vi "CSM - State Table - DebugTool.vi"() -> ()   [LabVIEW 2014]
uses:
  _Support/Typedef/_CSM_GlobalLog_MSG.ctl
  _Support/Typedef/_CSM_GlobalLog_MSG_TYPE.ctl
  _Polymophic/Add State(s) to Queue By BOOL(Element).vi
  _Support/GlobalEvent/FGV-GlobalEventRef.vi
  <resource>/dialog/lvconfig.llb/LV Config Write Numeric (I32).vi
  <resource>/dialog/lvconfig.llb/LV Config Read Numeric (I32).vi
  _Support/csm-tool-support.lvlib
  Communicable State Machine.lvlib
panel:
  in  "Clear JKISM":bool
  out "Dashboard":T1(array[cluster])
  out "Table Control":string[][](table)
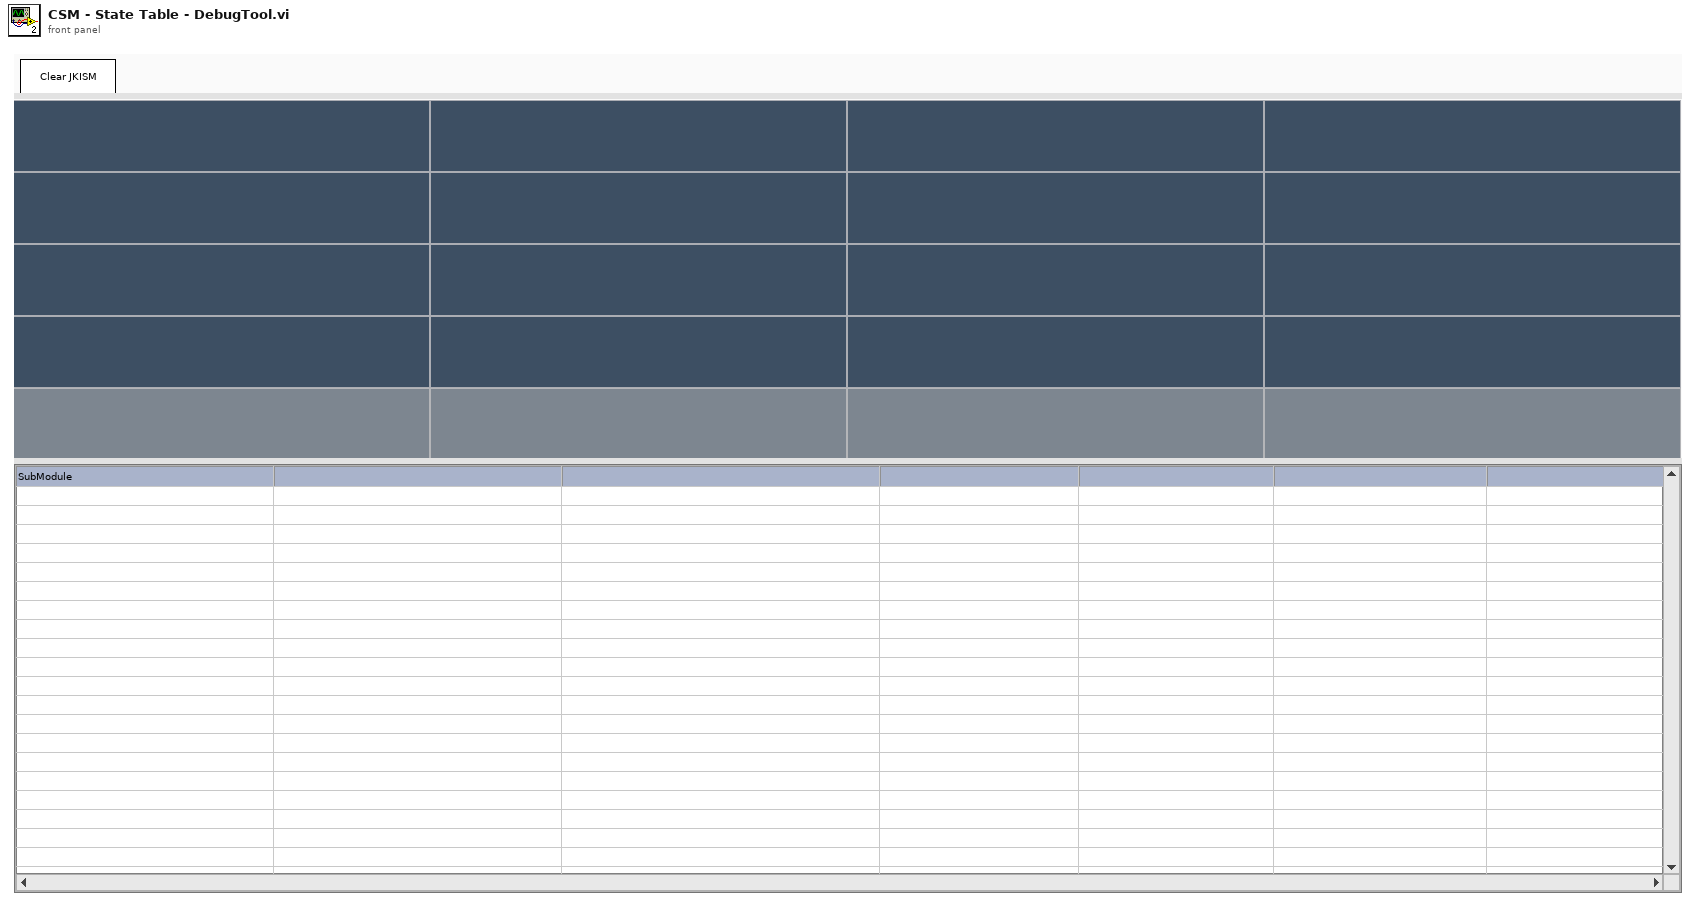
[diagram p1: front panel]
types:
  T1 = cluster{"Label":string, "Value":string, "String":string}[][]
  T2 = enum32{"Invalid", "Standard", "Closed", "Hidden", "Minimized", "Maximized"}
  T3 = enum32{"invalid app kind", "Development System", "Run Time System", "Student Edition", "Embedded LabVIEW", "Evaluation", "Custom"}
  T4 = typedef "Communicable State Machine.lvlib/_CSM_GlobalLog_MSG.ctl" = cluster{"Name(\"\" to use uuid)":string, "Current State":string, "Arguments":string, "Argument - State":string, "From Who":string, "Complete(T)/Start(F)":bool, "Type":T5}
  T5 = typedef "Communicable State Machine.lvlib/_CSM_GlobalLog_MSG_TYPE.ctl" = enum16{"User Log", "State Change", "Status", "Interrupt", "Register", "Unregister"}
  T6 = cluster{"Label":string, "Value":string, "String":string}
  T7 = cluster{"Core":cluster{"Current VI Reference":refnum<vi>, "Close Panel on Exit?":bool}, "Global-DataTable":string[][], "NumCols":i16, "NumRows":i16, "CSM Global Log Event":refnum<user-event>, "Log":T4, "JKISM Names":string[]}
  T8 = cluster{"Current VI Reference":refnum<vi>, "Close Panel on Exit?":bool}
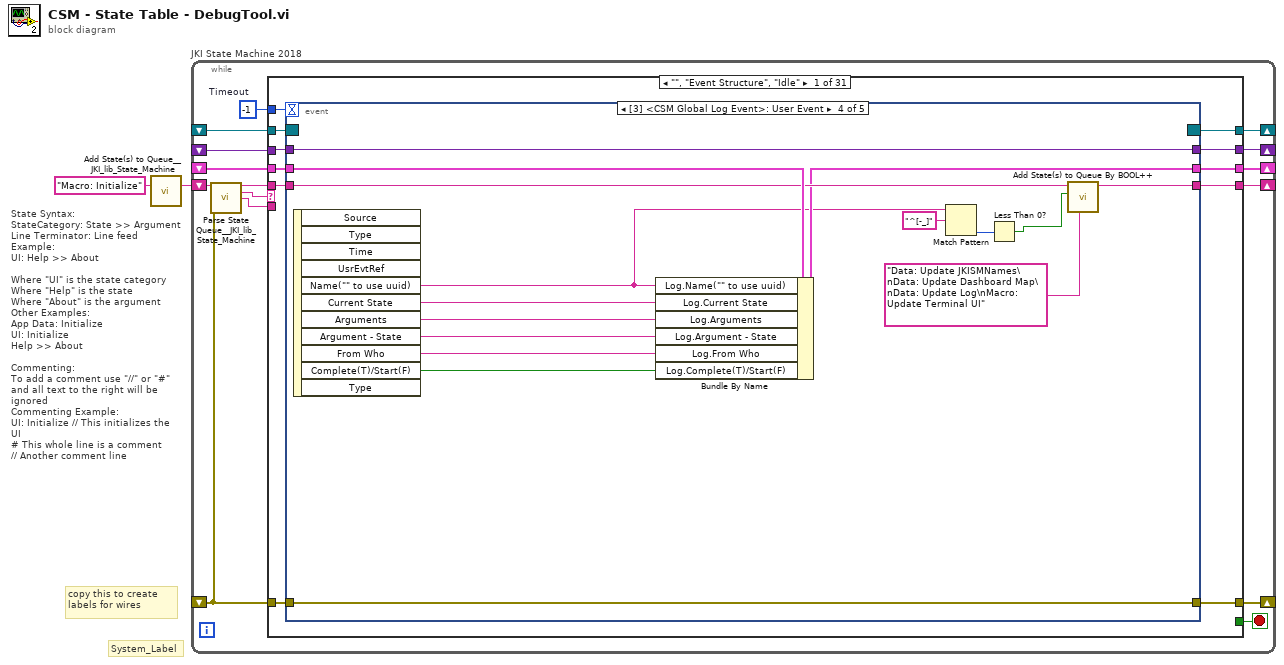
[diagram p0: block diagram]
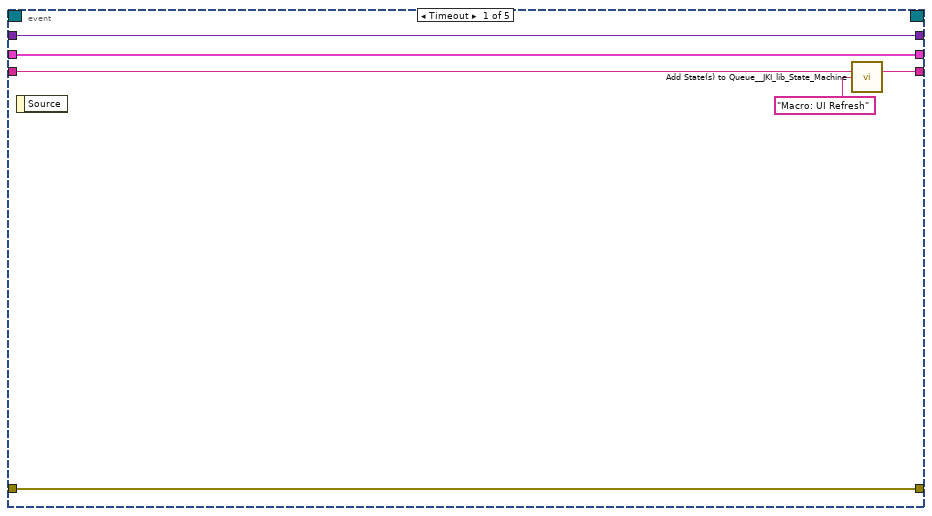
[diagram p2: hidden frame]
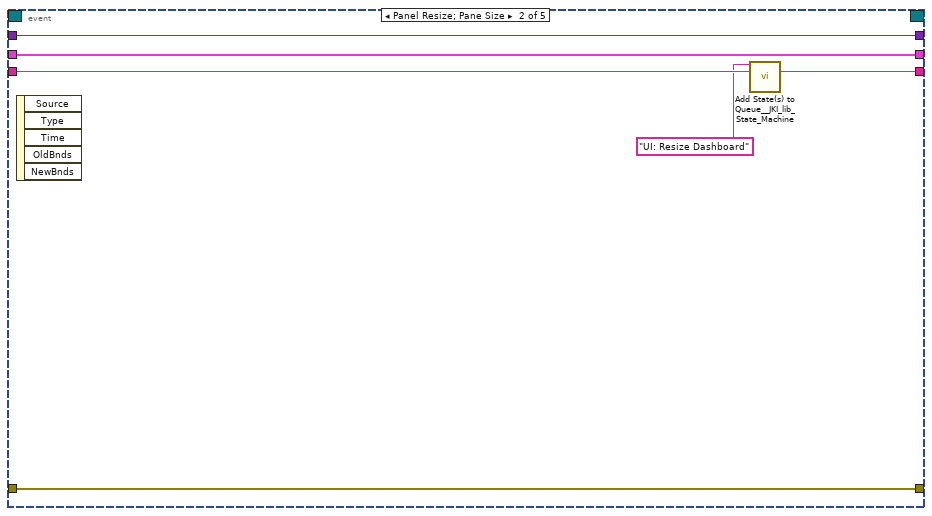
[diagram p3: hidden frame]
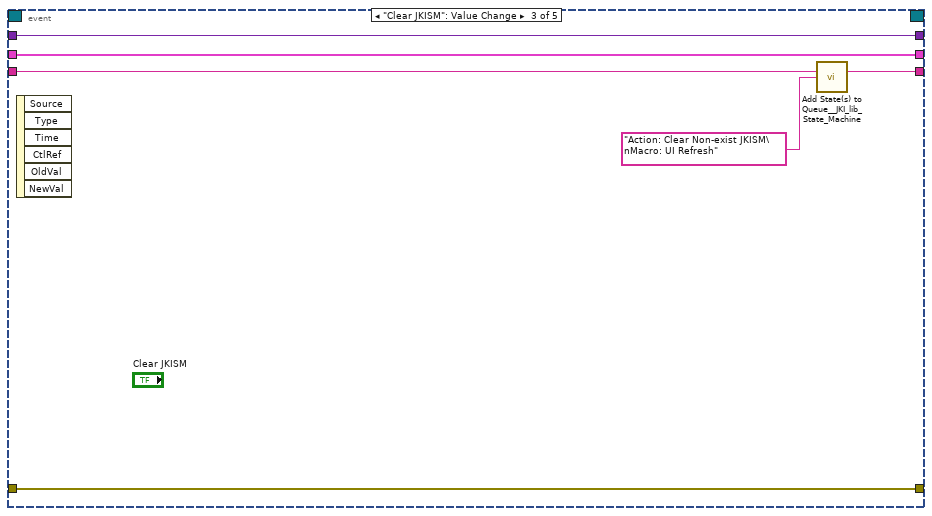
[diagram p4: hidden frame]
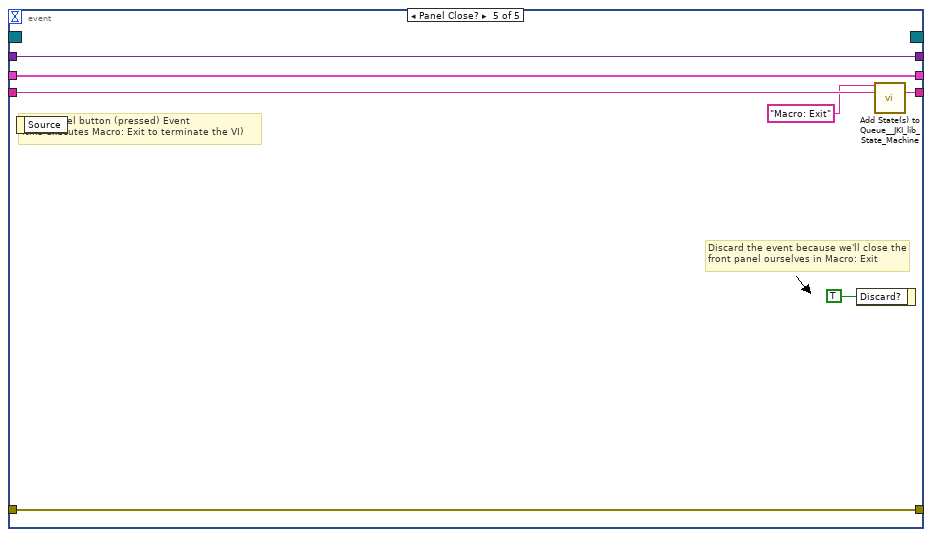
[diagram p5: hidden frame]
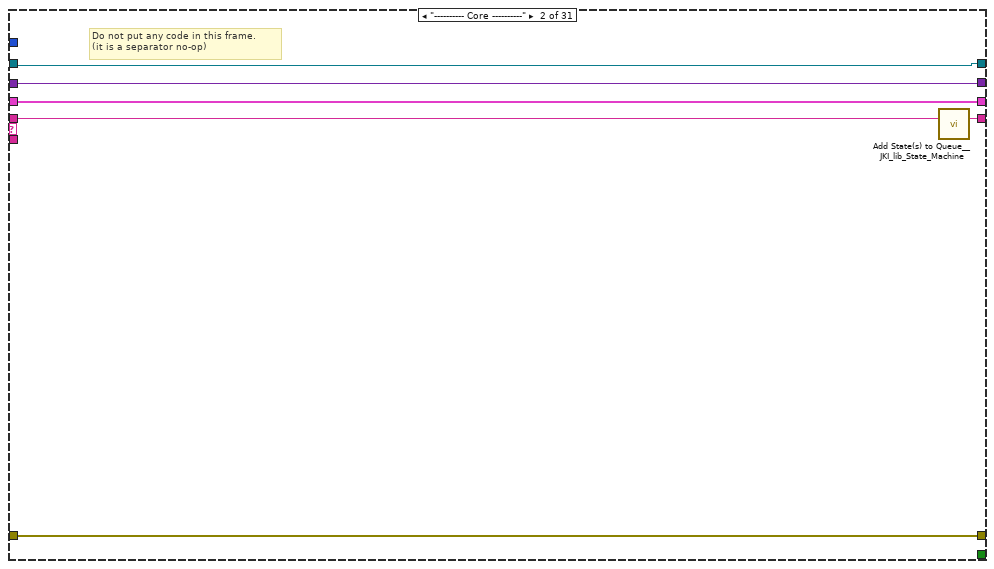
[diagram p6: hidden frame]
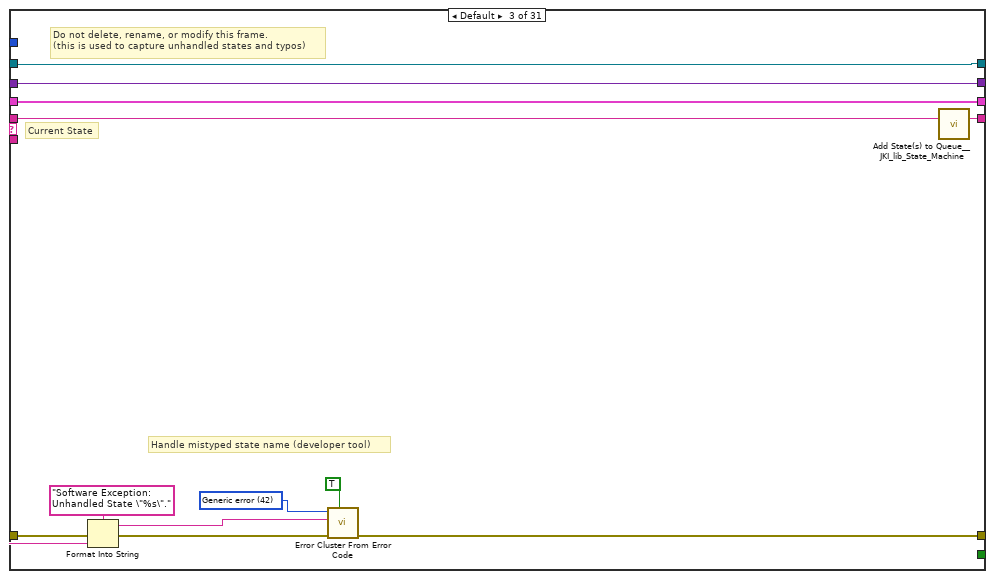
[diagram p7: hidden frame]
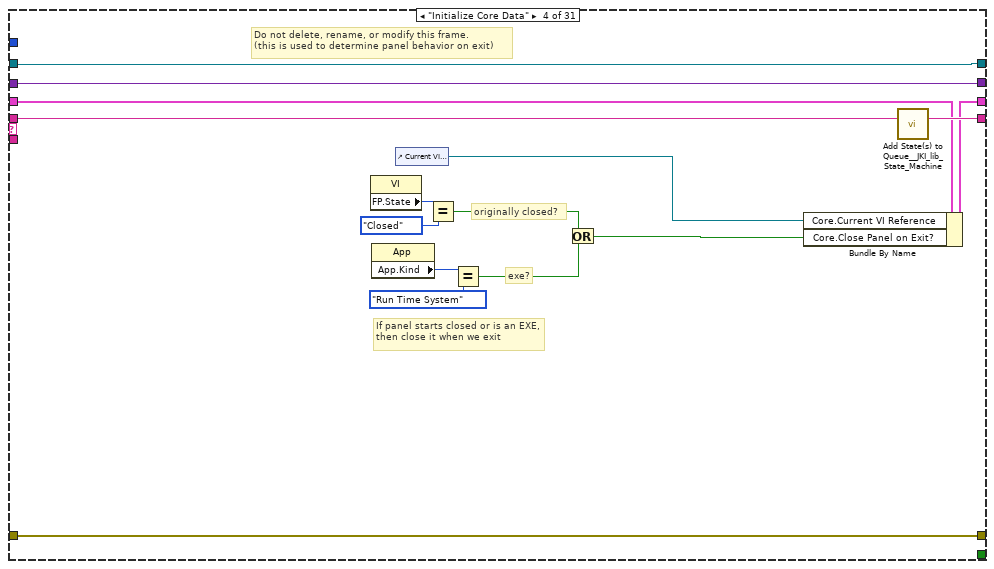
[diagram p8: hidden frame]
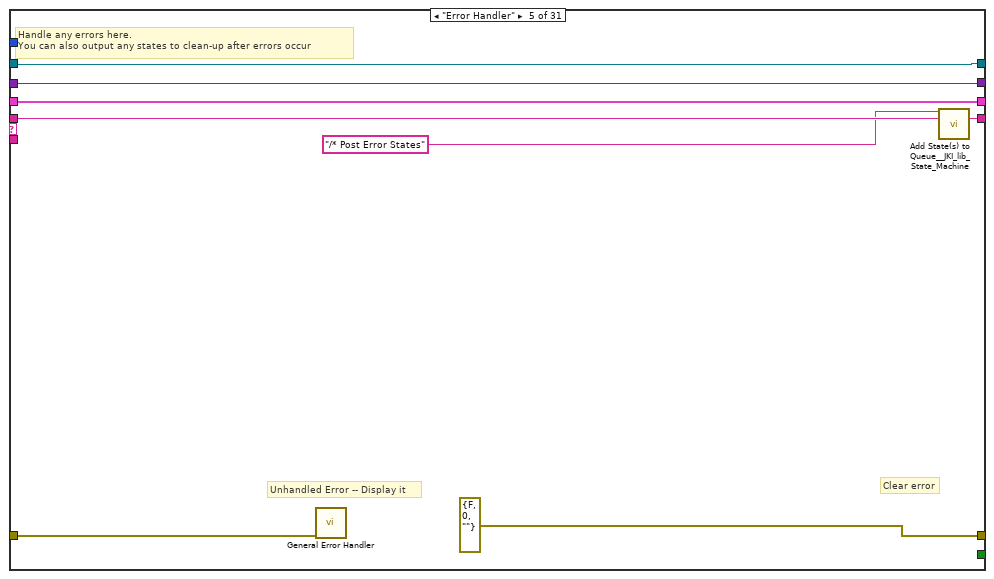
[diagram p9: hidden frame]
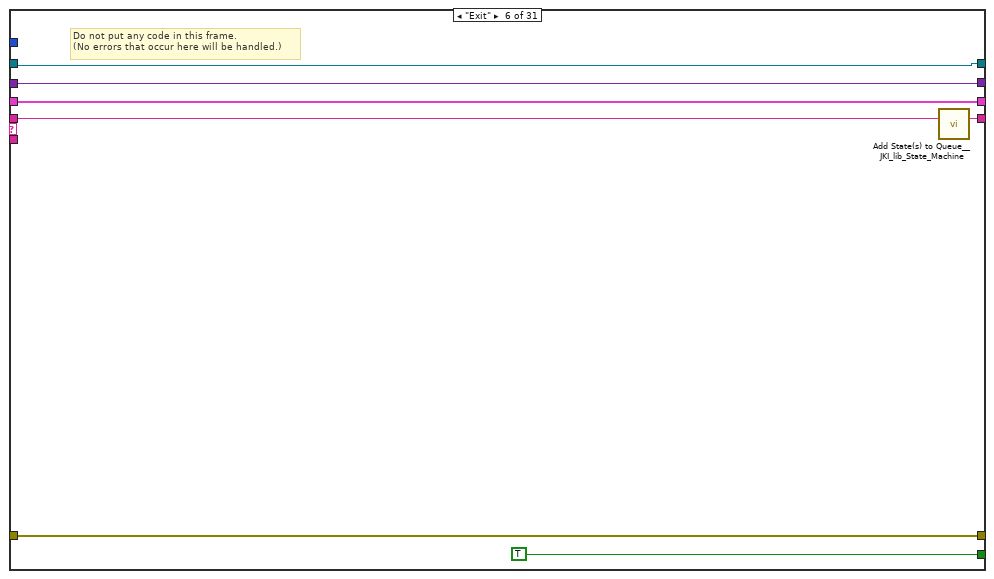
[diagram p10: hidden frame]
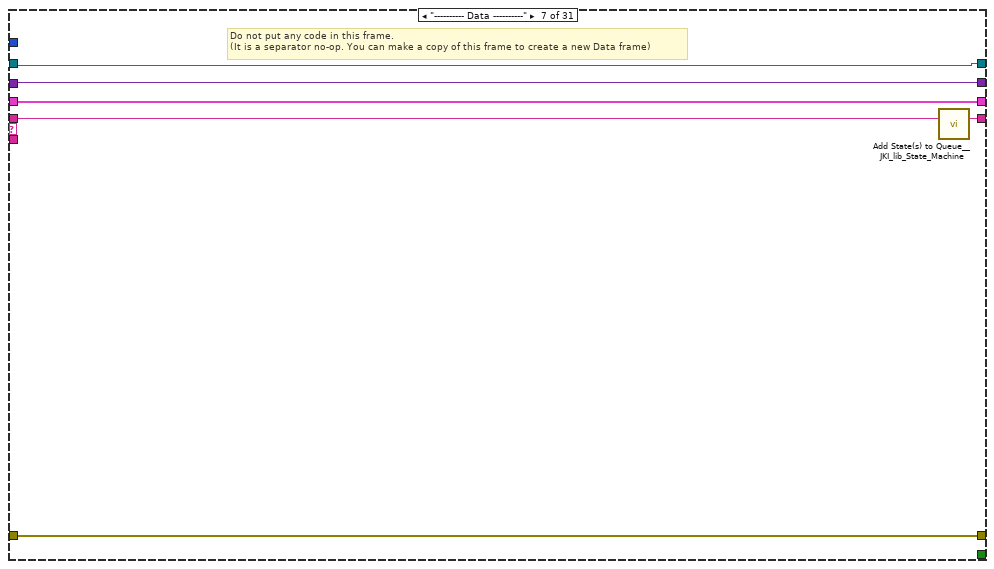
[diagram p11: hidden frame]
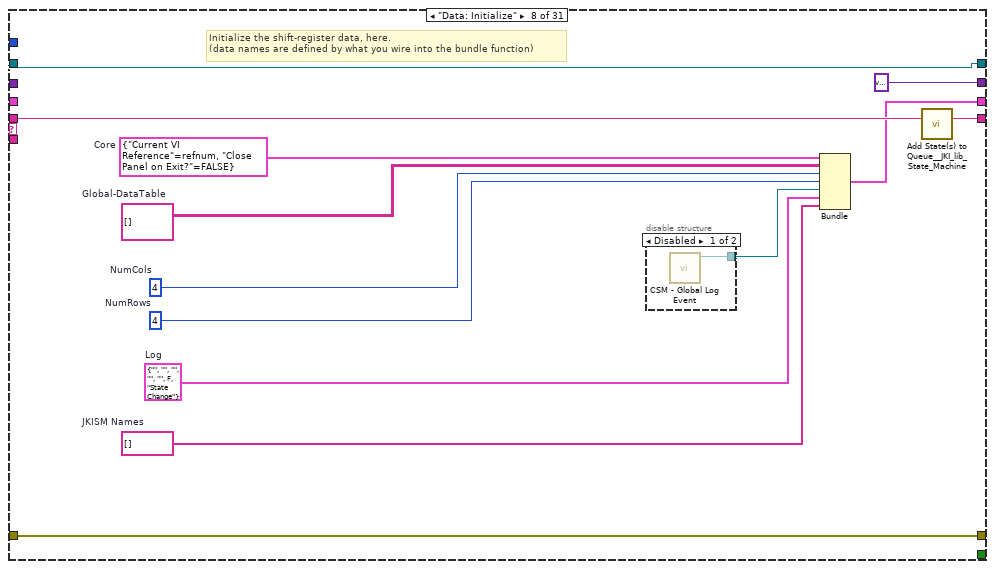
[diagram p12: hidden frame]
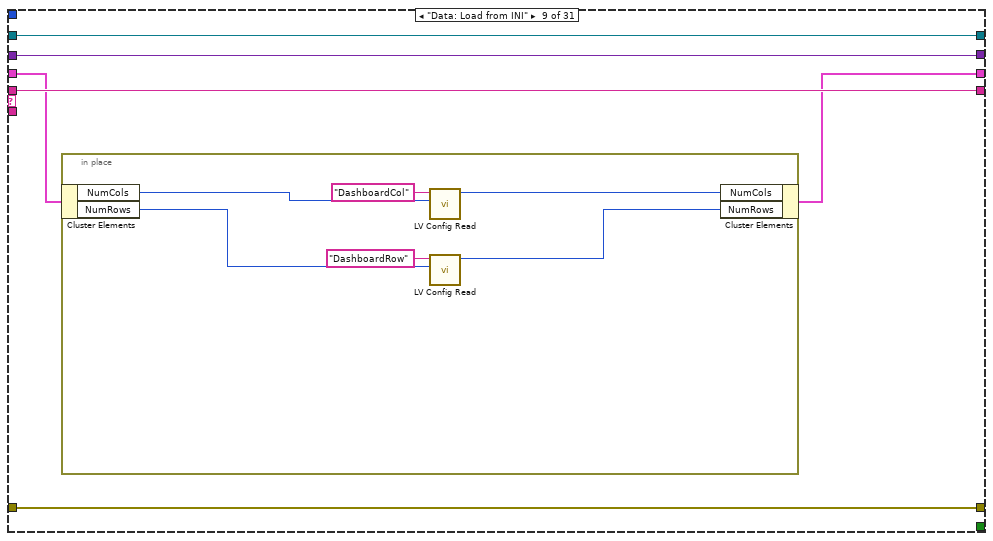
[diagram p14: hidden frame]
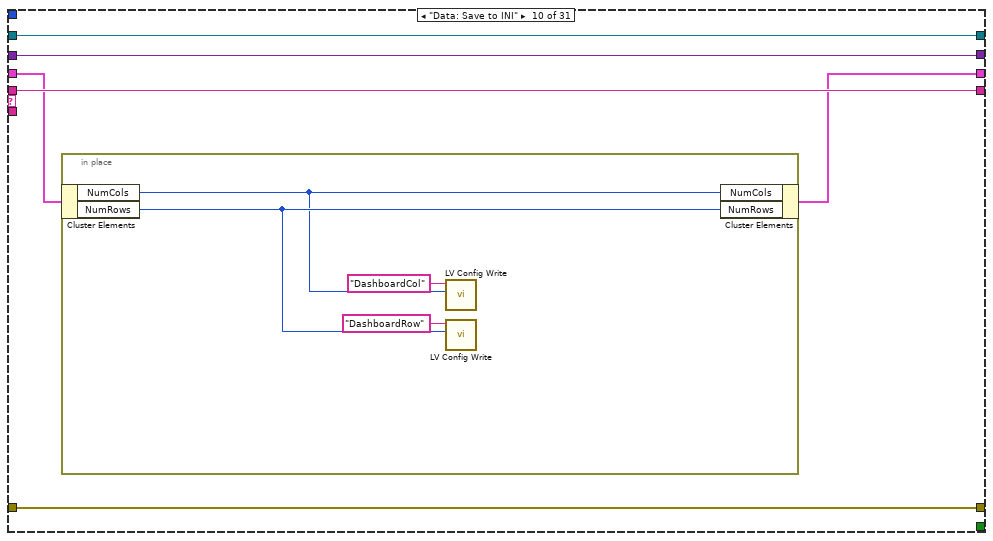
[diagram p15: hidden frame]
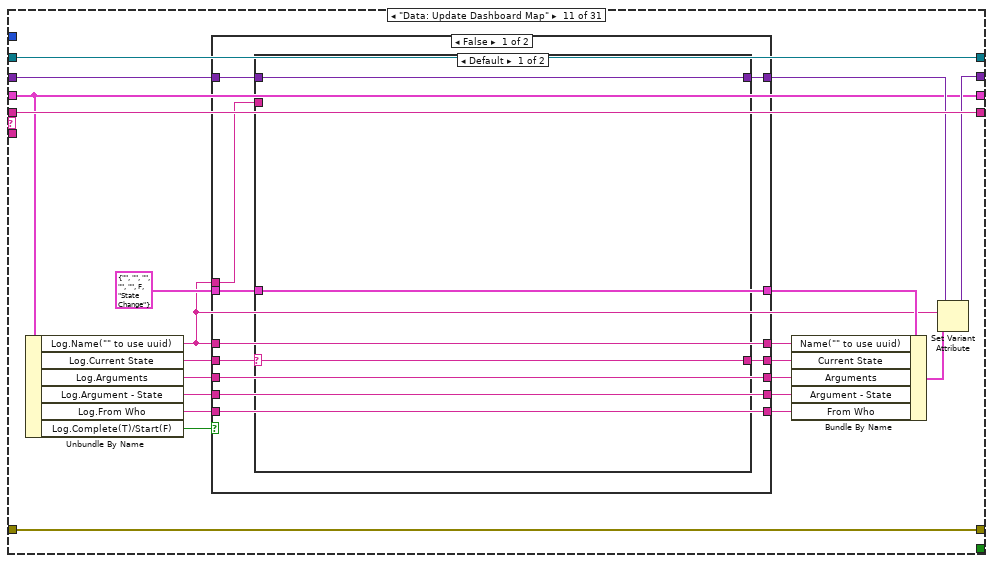
[diagram p16: hidden frame]
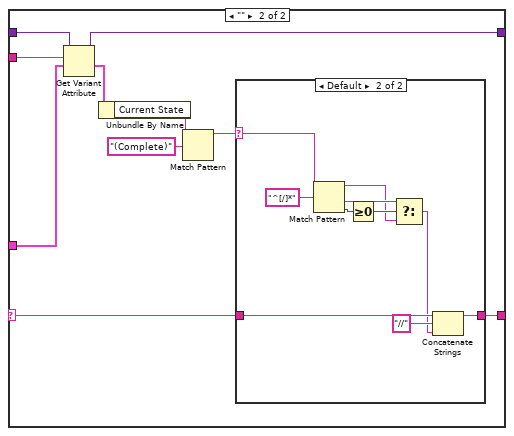
[diagram p17: hidden frame]
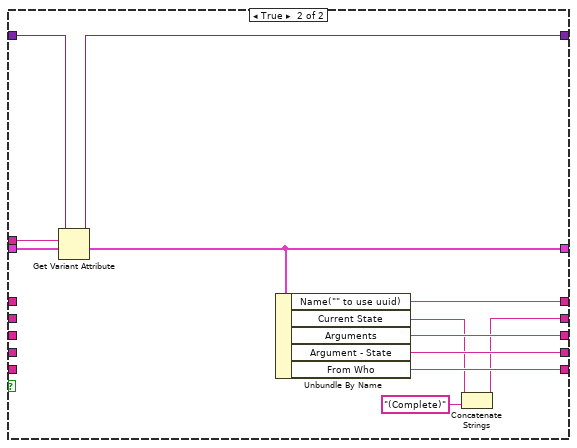
[diagram p19: hidden frame]
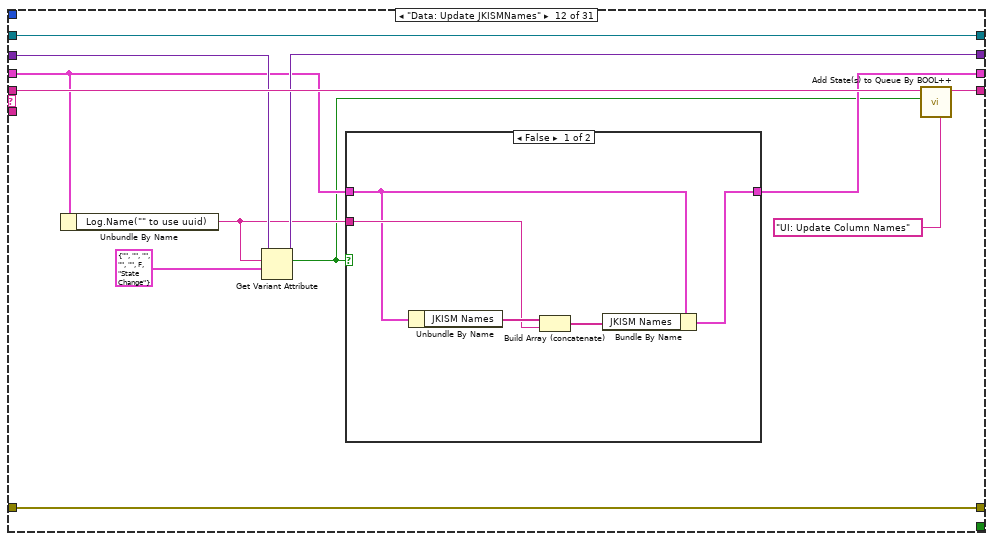
[diagram p20: hidden frame]
diagram:
  # "State Syntax:\nStateCategory: State >> Argument\nLine Terminator: Line feed\nExample:\nUI: Help >> About\n\nWhere \"UI\" is the state category\nWhere \"Help\" is the state\nWhere \"About\" is the argument\nOther Examples:\nApp Data: Initialize\nUI: Initialize\nHelp >> About\n\nCommenting:\nTo add a comment use \"//\" or \"#\" and all text to the right will be ignored\nCommenting Example:\nUI: Initialize // This initializes the UI\n# This whole line is a comment\n// Another comment line"
  # "copy this to create labels for wires"
  # "System_Label"
  n1 = call <vilib>:"Add State(s) to Queue__JKI_lib_State_Machine.vi"("State(s) in (\"\")"="Macro: Initialize") -> ("States Out"=w1:string)  [unwired: 14 in]
  n2 = while "JKI State Machine 2018" {
    shift-right: [w10] -> _
    shift-left: _ -> [w9]
    shift-right: [w13] -> _
    shift-left: _ -> [w7]
    shift-right: [w12] -> _
    shift-left: w1 -> [w14]
    shift-right: [w6] -> _
    shift-left: _ -> [w5]
    shift-right: [w4] -> _
    shift-left: _ -> [w3]
    stop <- w11 stop-if-true
    w8 = -1  # Timeout
    n3 = call <vilib>:"Parse State Queue__JKI_lib_State_Machine.vi"("State Queue"=w14, "Error In (no error)"=w7) -> ("Remaining States"=w16:string, "Current State"=w17:string, "Arguments"=w15:string)  [unwired: 11 in]
    n4 = case shown="\"\", \"Event Structure\", \"Idle\"" w17 {
      selector: w17 -> [_ _ w78 _ _ _ _ _ _ _ _ _ _ _ _ _ _ _ _ _ _ _ _ _ _ _ _ _ _ _ _]
      tunnel: w16 -> [w28 w75 w82 w103 w111 w118 w124 w137 w143 w155 w180 w237 w260 w283 w289 w298 w310 w323 w400 w415 w426 w431 w439 w447 w454 w461 w469 w476 w489 w493 w504]
      tunnel: w15 -> [_ _ _ _ _ _ _ _ _ _ _ _ _ _ _ _ w305 w317 _ _ _ _ _ _ _ _ _ _ _ _ _]
      tunnel: w9 -> [w26 w72 w80 w96 w108 w116 w121 _ w142 w154 w167 w231 w256 w278 w286 w294 w308 w319 w396 w412 w423 w430 w438 w443 w451 w458 w464 w473 w486 w492 w503]
      tunnel: [w25 w73 w84 w100 errorcluster {"status"=FALSE, "code"=0, "source"=""} ("error out") w115 w122 w133 w144 w156 w181 w238 w261 w277 w287 w296 w306 w320 w397 w413 w427 w432 w440 w448 w452 w459 w467 w474 w487 w494 w505] -> w13
      tunnel: w7 -> [w24 w73 w83 w100 w107 w115 w122 w133 w144 w156 w181 w238 w261 w280 w287 w296 w307 w321 _ w413 w427 w432 w440 w448 w452 w459 w467 w474 w487 w494 w505]
      tunnel: [w27 w74 w81 w102 w110 w117 w123 w136 w143 w155 w180 w229 w260 w282 w288 w297 w309 w322 w399 w414 w426 w431 w439 w447 w453 w460 w468 w475 w488 w493 w504] -> w12
      tunnel: [_ _ _ _ _ TRUE _ _ _ _ _ _ _ _ _ _ _ _ _ _ _ _ _ _ _ _ _ _ _ _ _] -> w11
      tunnel: [w23 w72 w80 w101 w108 w116 w121 w135 w141 w153 w167 w230 w256 w278 w286 w294 w308 w319 w396 w412 w423 w430 w434 w443 w451 w458 w464 w473 w486 w492 w503] -> w10
      tunnel: w8 -> [w22 _ _ _ _ _ _ _ _ _ _ _ _ _ _ _ _ _ _ _ _ _ _ _ _ _ _ _ _ _ _]
      tunnel: [w20 w71 w77 w90 w105 w113 w120 variant w140 w152 w168 w235 w257 w276 w285 w291 w304 w316 w393 w407 w425 w429 w437 w446 w450 w456 w463 w471 w479 w491 w499] -> w6
      tunnel: w5 -> [w21 w71 w77 w90 w105 w113 w120 _ w140 w152 w169 w233 w258 w276 w285 w291 w304 w316 w393 w406 w425 w429 w437 w446 w450 w456 w463 w471 w479 w491 w501]
      tunnel: [w18 w70 w76 w89 w104 w112 w119 w128 w139 w151 w179 w236 w259 w275 w284 w290 w303 w315 w392 w403 w424 w428 w435 w445 w449 w455 w462 w470 w478 w490 w502] -> w4
      tunnel: w3 -> [w19 w70 w76 w89 w104 w112 w119 w128 w139 w151 w179 w236 w259 w275 w284 w290 w303 w315 w392 w403 w424 w428 _ w445 w449 w455 w462 w470 w478 w490 w502]
      frame "", "Event Structure", "Idle" {
        n5 = event shown="[3] <CSM Global Log Event>: User Event" {
          selector: w19 -> [_ _ _ _ _]
          dyn-events: [_ _ _ _ _] -> w18
          timeout: w22 -> [_ _ _ _ _]
          tunnel: w28 -> [w34 w37 w43 w57 w69]
          tunnel: [w33 w38 w42 w61 w68] -> w27
          tunnel: w26 -> [w31 w39 w45 w58 w67]
          tunnel: [w32 w40 w46 w62 w64] -> w25
          tunnel: w24 -> [w32 w40 w46 w62 w64]
          tunnel: [w31 w39 w45 w56 w67] -> w23
          tunnel: w21 -> [w29 w35 w44 w59 w63]
          tunnel: [w29 w35 w44 w59 w63] -> w20
          event Timeout {
            n6 = event-data() -> ()  [unwired: 1 in, 1 out]
            n7 = call <vilib>:"Add State(s) to Queue__JKI_lib_State_Machine.vi"("State(s) in (\"\")"=w34, "State(s) at Back (\"\")"="Macro: UI Refresh" ("State(s) in Front (\"\")")) -> ("States Out"=w33:string)  [unwired: 13 in]
          }
          event Panel Resize; Pane Size {
            n8 = event-data() -> ()  [unwired: 1 in, 5 out]
            n9 = call <vilib>:"Add State(s) to Queue__JKI_lib_State_Machine.vi"("State(s) in Front (\"\")"="UI: Resize Dashboard" ("State(s) in Front (\"\")"), "State(s) in (\"\")"=w37) -> ("States Out"=w38:string)  [unwired: 13 in]
          }
          event "Clear JKISM": Value Change {
            n10 = event-data() -> ()  [unwired: 1 in, 6 out]
            n11 = call <vilib>:"Add State(s) to Queue__JKI_lib_State_Machine.vi"("State(s) in (\"\")"=w43, "State(s) at Back (\"\")"="Action: Clear Non-exist JKISM\nMacro: UI Refresh" ("State(s) at Back (\"\")")) -> ("States Out"=w42:string)  [unwired: 13 in]
          }
          event User Event {
            n12 = event-data() -> ("Name(\"\" to use uuid)"=w50:string, "Current State"=w51:string, "Arguments"=w52:string, "Argument - State"=w53:string, "From Who"=w54:string, "Complete(T)/Start(F)"=w55:bool)  [unwired: 1 in, 5 out]
            n13 = Bundle By Name(cluster=w58, "Log.Name(\"\" to use uuid)"=w50, "Log.Current State"=w51, "Log.Arguments"=w52, "Log.Argument - State"=w53, "Log.From Who"=w54, "Log.Complete(T)/Start(F)"=w55) -> (w56:T7)
            n14 = Match Pattern(string=w50, regular expression="^[-_]") -> (offset past match=w48:i32)  [unwired: 1 in, 3 out]
            n15 = Less Than 0?(x=w48) -> (x < 0?=w47:bool)
            n16 = call-poly "Add State(s) to Queue By BOOL++.vi"("TRUE(\"\")"="Data: Update JKISMNames\nData: Update Dashboard Map\nData: Update Log\nMacro: Update Terminal UI" ("State(s) at Back (\"\")"), "Bool"=w47, "State Queue(\"\")"=w57) -> ("State Queue Out"=w61:string)  [unwired: 8 in]
          }
          event Panel Close? {
            # "Discard the event because we'll close the front panel ourselves in Macro: Exit"
            # "Close Panel button (pressed) Event\n(this executes Macro: Exit to terminate the VI)"
            n17 = event-data() -> ()  [unwired: 1 in, 1 out]
            n18 = event-data("Discard?"=TRUE) -> ()  [unwired: 1 in, 1 out]
            n19 = call <vilib>:"Add State(s) to Queue__JKI_lib_State_Machine.vi"("State(s) in Front (\"\")"="Macro: Exit", "State(s) in (\"\")"=w69) -> ("States Out"=w68:string)  [unwired: 13 in]
          }
        }
      }
      frame "---------- Core ----------" {
        # "Do not put any code in this frame.\n(it is a separator no-op)"
        n20 = call <vilib>:"Add State(s) to Queue__JKI_lib_State_Machine.vi"("State(s) in (\"\")"=w75) -> ("States Out"=w74:string)  [unwired: 14 in]
      }
      frame Default {
        w87 = 42 items=["No error", "Argument error", "Memory is full", "Out of zone", "End of file", "File already open", "Generic file I/O error", "File not found", "File permission error", "Disk is full", "Duplicate path", "Too many files open", "System feature not enabled", "Resource file not found", "Cannot add resource", "Resource not found", "Image not found", "Image memory error", "Pen does not exist", "Config type invalid", "Config token not found", "Config parse error", "Config memory error", "Bad external code format", "Bad external code offset", "External code not present", "Null window", "Destroy window error", "Null menu", "Print aborted", "Bad print record", "Print driver error", "Windows error during printing", "Memory error during printing", "Print dialog error", "Generic print error", "Invalid device refnum", "Device not found", "Device parameter error", "Device unit error", "Cannot open device", "Device call aborted", "Generic error", "Cancelled by user", "Object ID too low", "Object ID too high", "Object not in heap", "Unknown heap", "Unknown object (invalid DefProc)", "Unknown object (DefProc not in table)", "Message out of range", "Invalid (null) method", "Unknown message", "Manager call not supported", "Bad address", "Network operation in progress", "Network operation timed out", "Connection is busy", "Network attribute not supported", "Network error", "Address in use", "System out of memory", "Connection aborted", "Connection refused", "Not connected", "Already connected", "Connection closed", "Initialization error (interapplication manager)", "Bad occurrence", "Wait on unbound occurrence handler", "Occurrence queue overflow", "Datalog type conflict", "Unused", "Unrecognized type (interapplication manager)", "Memory corrupt", "Failed to make temporary DLL", "Old CIN version", "Drag socket not found", "Failed to load drop-object", "Failed to register OLE object", "Failed to release OLE object", "Format specifier type mismatch", "Unknown format specifier", "Too few format specifiers", "Too many format specifiers", "Scan failed", "Newer CIN version", "Error converting to variant", "Runtime menu error", "Password tampered", "Variant attribute not found", "Incompatible variant data type", "Event data is not available", "Event Store is not present", "Occurrence is not found", "Event Queue is not created", "Event info is not available", "Refnum passed is NULL", "Error retrieving Class GUID", "Error retrieving CoClass GUID", "Error retrieving TypeLib GUID.", "Bad built application magic bytes.", "Specific driver is different from the specific driver associated with the Logical Name.", "There is no session opened to the class driver.", "Max Error", "MAX - Error with config objects", "MAX - Error loading configuration", "MAX - Group not supported"]
        # "Current State"
        # "Do not delete, rename, or modify this frame.\n(this is used to capture unhandled states and typos)"
        # "Handle mistyped state name (developer tool)"
        n21 = Format Into String(format string="Software Exception: Unhandled State \"%s\"." ("message"), error in=w83, w78) -> (resulting string=w86:string, error out=w85:errorcluster)  [unwired: 1 in]
        n22 = call <vilib>:"Error Cluster From Error Code.vi"("show call chain? (False)"=TRUE, "error in (no error)"=w85, "error message (\"\")"=w86, "error code (0)"=w87) -> ("error out"=w84:errorcluster)  [unwired: 5 in]
        n23 = call <vilib>:"Add State(s) to Queue__JKI_lib_State_Machine.vi"("State(s) in (\"\")"=w82) -> ("States Out"=w81:string)  [unwired: 14 in]
      }
      frame "Initialize Core Data" {
        # "Do not delete, rename, or modify this frame.\n(this is used to determine panel behavior on exit)"
        # "originally closed?"
        # "exe?"
        # "If panel starts closed or is an EXE, then close it when we exit"
        n24 = property class="VI"() -> ("FP.State"=w93:T2)  [unwired: 2 in, 2 out]
        n25 = property class="App"() -> ("App.Kind"=w99:T3)  [unwired: 2 in, 2 out]
        n26 = control-ref of="Current VI Reference"() -> (w94:refnum<vi>)
        n27 = Equal?(x=w93, y=T2."Closed" ("Front Panel Window:State")) -> (x = y?=w91:bool)
        n28 = Equal?(x=w99, y=T3."Run Time System" ("Application:Kind")) -> (x = y?=w97:bool)
        n29 = Or(x=w91, y=w97) -> (x .or. y?=w95:bool)
        n30 = Bundle By Name(cluster=w96, "Core.Current VI Reference"=w94, "Core.Close Panel on Exit?"=w95) -> (w101:T7)
        n31 = call <vilib>:"Add State(s) to Queue__JKI_lib_State_Machine.vi"("State(s) in (\"\")"=w103) -> ("States Out"=w102:string)  [unwired: 14 in]
      }
      frame "Error Handler" {
        # "Unhandled Error -- Display it"
        # "Handle any errors here.\nYou can also output any states to clean-up after errors occur"
        # "Clear error"
        n32 = call <vilib>:"General Error Handler.vi"("error in (no error)"=w107) -> ()  [unwired: 10 in, 5 out]
        n33 = call <vilib>:"Add State(s) to Queue__JKI_lib_State_Machine.vi"("State(s) in Front (\"\")"="/* Post Error States", "State(s) in (\"\")"=w111) -> ("States Out"=w110:string)  [unwired: 13 in]
      }
      frame "Exit" {
        # "Do not put any code in this frame.\n(No errors that occur here will be handled.)"
        n34 = call <vilib>:"Add State(s) to Queue__JKI_lib_State_Machine.vi"("State(s) in (\"\")"=w118) -> ("States Out"=w117:string)  [unwired: 14 in]
      }
      frame "---------- Data ----------" {
        # "Do not put any code in this frame.\n(It is a separator no-op. You can make a copy of this frame to create a new Data frame)"
        n35 = call <vilib>:"Add State(s) to Queue__JKI_lib_State_Machine.vi"("State(s) in (\"\")"=w124) -> ("States Out"=w123:string)  [unwired: 14 in]
      }
      frame "Data: Initialize" {
        w125 = string[] []  # JKISM Names
        w126 = T4 {"Name(\"\" to use uuid)"="", "Current State"="", "Arguments"="", "Argument - State"="", "From Who"="", "Complete(T)/Start(F)"=FALSE, "Type"=enum."State Change"}  # Log
        w131 = i16 4  # NumCols
        w130 = i16 4  # NumRows
        w132 = string[][] []  # Global-DataTable
        w134 = T8 {"Current VI Reference"=refnum, "Close Panel on Exit?"=FALSE}  # Core
        # "Initialize the shift-register data, here.\n(data names are defined by what you wire into the bundle function)"
        n36 = disable-structure shown="Disabled" {
          disable-tunnel: [w138 _] -> w127
          frame Disabled {
            n37 = call "CSM - Global Log Event.vi"() -> ("CSM Global Log Event"=w138:refnum<user-event>)  [unwired: 10 in, 1 out]
          }
          frame Enabled {
          }
        }
        n38 = Bundle("Core"=w134, "Global-DataTable"=w132, "NumCols"=w131, "NumRows"=w130, "CSM Global Log Event"=w127, "Log"=w126, "JKISM Names"=w125) -> (w135:T7)  [unwired: 1 in]
        n39 = call <vilib>:"Add State(s) to Queue__JKI_lib_State_Machine.vi"("State(s) in (\"\")"=w137) -> ("States Out"=w136:string)  [unwired: 14 in]
      }
      frame "Data: Load from INI" {
        n40 = in-place {
          n41 = in-place-cluster #1(w142) -> ("NumCols"=w146:i16, "NumRows"=w149:i16)
          n42 = call-poly <resource>:"LV Config Read.vi"("default value"=w146, "key"="DashboardCol") -> ("value"=w145:i32)  [unwired: 3 in, 2 out]
          n43 = call-poly <resource>:"LV Config Read.vi"("default value"=w149, "key"="DashboardRow") -> ("value"=w148:i32)  [unwired: 3 in, 2 out]
          n44 = in-place-cluster #1("NumCols"=w145, "NumRows"=w148) -> (w141:T7)
        }
      }
      frame "Data: Save to INI" {
        n45 = in-place {
          n46 = in-place-cluster #2(w154) -> ("NumCols"=w157:i16, "NumRows"=w158:i16)
          n47 = call-poly <resource>:"LV Config Write.vi"("value"=w157, "key"="DashboardCol") -> ()  [unwired: 5 in, 1 out]
          n48 = call-poly <resource>:"LV Config Write.vi"("value"=w158, "key"="DashboardRow") -> ()  [unwired: 5 in, 1 out]
          n49 = in-place-cluster #2("NumCols"=w157, "NumRows"=w158) -> (w153:T7)
        }
      }
      frame "Data: Update Dashboard Map" {
        n50 = Unbundle By Name(w167) -> ("Log.Name(\"\" to use uuid)"=w161:string, "Log.Current State"=w166:string, "Log.Arguments"=w165:string, "Log.Argument - State"=w164:string, "Log.From Who"=w163:string, "Log.Complete(T)/Start(F)"=w162:bool)
        n51 = case shown="False" w162 {
          tunnel: w169 -> [w187 w226]
          tunnel: [w186 w225] -> w177
          tunnel: T4 {"Name(\"\" to use uuid)"="", "Current State"="", "Arguments"="", "Argument - State"="", "From Who"="", "Complete(T)/Start(F)"=FALSE, "Type"=enum."State Change"} ("Cross JKI State Machine Data") -> [w184 w224]
          tunnel: w161 -> [w185 w223]
          tunnel: w163 -> [w191 _]
          tunnel: [w191 w222] -> w175
          tunnel: w164 -> [w190 _]
          tunnel: [w190 w221] -> w174
          tunnel: w165 -> [w189 _]
          tunnel: [w189 w220] -> w173
          tunnel: w166 -> [w183 _]
          tunnel: [w182 w215] -> w172
          tunnel: w161 -> [w188 _]
          tunnel: [w188 w217] -> w171
          tunnel: [w184 w218] -> w170
          frame False {
            n52 = case shown="Default" w183 {
              selector: w183 -> [w192 w195]
              tunnel: w187 -> [w193 w203]
              tunnel: [w193 w202] -> w186
              tunnel: w185 -> [_ w201]
              tunnel: w184 -> [_ w199]
              tunnel: [w192 w194] -> w182
              frame Default {
              }
              frame "" {
                n53 = Get Variant Attribute(Variant=w203, name=w201, default value (empty Variant)=w199) -> (duplicate Variant=w202:variant, value=w200:T4)  [unwired: 1 in, 2 out]
                n54 = Unbundle By Name(w200) -> ("Current State"=w198:string)
                n55 = Match Pattern(string=w198, regular expression="(Complete)") -> (before substring=w196:string)  [unwired: 1 in, 3 out]
                n56 = case shown="Default" w196 {
                  selector: w196 -> [_ w210]
                  tunnel: w195 -> [w204 w214]
                  tunnel: [w204 w213] -> w194
                  frame "" {
                  }
                  frame Default {
                    n57 = Match Pattern(string=w210, regular expression="^[/]*") -> (before substring=w205:string, after substring=w207:string, offset past match=w209:i32)  [unwired: 1 in, 1 out]
                    n58 = Greater Or Equal To 0?(x=w209) -> (x >= 0?=w208:bool)
                    n59 = Select(t=w207, s=w208, f=w205) -> (s? t:f=w206:string)
                    n60 = Concatenate Strings(w214, "//" ("string"), w206) -> (w213:string)
                  }
                }
              }
            }
          }
          frame True {
            n61 = Get Variant Attribute(Variant=w226, name=w223, default value (empty Variant)=w224) -> (duplicate Variant=w225:variant, value=w218:T4)  [unwired: 1 in, 2 out]
            n62 = Unbundle By Name(w218) -> ("Name(\"\" to use uuid)"=w217:string, "Current State"=w216:string, "Arguments"=w220:string, "Argument - State"=w221:string, "From Who"=w222:string)
            n63 = Concatenate Strings(w216, "(Complete)" ("string")) -> (w215:string)
          }
        }
        n64 = Bundle By Name(cluster=w170, "Name(\"\" to use uuid)"=w171, "Current State"=w172, "Arguments"=w173, "Argument - State"=w174, "From Who"=w175) -> (w178:T4)
        n65 = Set Variant Attribute(Variant=w177, name=w161, value=w178) -> (Variant out=w168:variant)  [unwired: 1 in, 2 out]
      }
      frame "Data: Update JKISMNames" {
        n66 = Unbundle By Name(w231) -> ("Log.Name(\"\" to use uuid)"=w232:string)
        n67 = Get Variant Attribute(Variant=w233, name=w232, default value (empty Variant)=T4 {"Name(\"\" to use uuid)"="", "Current State"="", "Arguments"="", "Argument - State"="", "From Who"="", "Complete(T)/Start(F)"=FALSE, "Type"=enum."State Change"} ("Cross JKI State Machine Data")) -> (duplicate Variant=w235:variant, found=w228:bool)  [unwired: 1 in, 2 out]
        n68 = case shown="False" w228 {
          tunnel: w231 -> [w241 w244]
          tunnel: w232 -> [w242 _]
          tunnel: [w239 w244] -> w230
          frame False {
            n69 = Unbundle By Name(w241) -> ("JKISM Names"=w243:string[])
            n70 = Build Array (concatenate)(w243, w242) -> (w240:string[])
            n71 = Bundle By Name(cluster=w241, "JKISM Names"=w240) -> (w239:T7)
          }
          frame True {
          }
        }
        n72 = call-poly "Add State(s) to Queue By BOOL++.vi"("False(\"\")"="UI: Update Column Names" ("TRUE(\"\")"), "Bool"=w228, "State Queue(\"\")"=w237) -> ("State Queue Out"=w229:string)  [unwired: 8 in]
      }
      frame "Data: Update Log" {
        n73 = Unbundle By Name(w256) -> ("JKISM Names"=w255:string[])
        n74 = for {
          shift-right: [w272] -> w257
          shift-left: w258 -> [w273]
          tunnel: w255 -> [w271] mode=indexing
          tunnel: [w269] -> w251 mode=indexing
          n75 = Get Variant Attribute(Variant=w273, name=w271, default value (empty Variant)=T4 {"Name(\"\" to use uuid)"="", "Current State"="", "Arguments"="", "Argument - State"="", "From Who"="", "Complete(T)/Start(F)"=FALSE, "Type"=enum."State Change"} ("Cross JKI State Machine Data")) -> (duplicate Variant=w272:variant, value=w270:T4)  [unwired: 1 in, 2 out]
          n76 = Unbundle By Name(w270) -> ("Current State"=w269:string)
        }
        n77 = Array Size(array=w251) -> (size(s)=w250:i32)
        n78 = feedback #3(string[][] []) -> (w249:string[][])
        n79 = Array Size(array=w249) -> (size(s)=w252:i32[])
        n80 = Index Array(array=w252) -> (element #1=w248:i32, element #2=w247:i32)  [unwired: 2 in]
        n81 = Greater?(x=w250, y=w247) -> (0:w245:bool)
        n82 = case shown="True" w245 {
          tunnel: w249 -> [w262 w268]
          tunnel: w248 -> [_ w266]
          tunnel: w247 -> [_ w264]
          tunnel: [w262 w263] -> w246
          frame False {
          }
          frame True {
            n83 = Initialize Array("" ("Current State"), w266) -> (w265:string[])
            n84 = Insert Into Array(array=w268, index (col)=w264, new element=w265) -> (w263:string[][])  [unwired: 1 in]
          }
        }
        n85 = Build Array (concatenate)(w251, w246) -> (w254:string[][])
        "Table Control" <- w254
        n86 = feedback-in #3(w254) -> ()
      }
      frame "Data: Cleanup" {
        # "Cleanup any data and references, here.\n(this is called automatically, by the Macro: Exit)"
        n87 = Unbundle By Name(w278) -> ("Core.Current VI Reference"=w281:refnum<vi>)
        n88 = Close Reference(reference=w281, error in (no error)=w280) -> (error out=w279:errorcluster)
        n89 = Merge Errors(w279) -> (w277:errorcluster)
        n90 = call <vilib>:"Add State(s) to Queue__JKI_lib_State_Machine.vi"("State(s) in (\"\")"=w283) -> ("States Out"=w282:string)  [unwired: 14 in]
      }
      frame "---------- UI ----------" {
        # "Do not put any code in this frame.\n(It is a separator no-op. You can make a copy of this frame to create a new UI frame)"
        n91 = call <vilib>:"Add State(s) to Queue__JKI_lib_State_Machine.vi"("State(s) in (\"\")"=w289) -> ("States Out"=w288:string)  [unwired: 14 in]
      }
      frame "UI: Initialize" {
        # "Initialize the User Interface, here.\n(this is called automatically, by the Macro: Init)"
        n92 = invoke class="VI" method="Default Vals.Reinit All"() -> (error out=w295:errorcluster)  [unwired: 3 in, 2 out]
        n93 = Unbundle By Name(w294) -> ("NumRows"=w293:i16, "NumCols"=w292:i16)
        n94 = flat-sequence {
          tunnel: w295 -> [_]
          tunnel: w293 -> [w300]
          tunnel: w292 -> [w299]
          frame #0 {
            n95 = Initialize Array(T6 {"Label"="", "Value"="", "String"=""} ("Dashboard"), w300, w299) -> (w301:T1)
            n96 = local write "Dashboard"(w301) -> ()
          }
        }
        n97 = call <vilib>:"Add State(s) to Queue__JKI_lib_State_Machine.vi"("State(s) in (\"\")"=w298) -> ("States Out"=w297:string)  [unwired: 14 in]
      }
      frame "UI: Cursor Set" {
        # "Argument"
        # "Set and Unset Cursor Busy.\n(Usage: \"UI: Cursor Set >> Busy|Idle\")"
        n98 = case shown="\"Idle\", Default" w305 {
          tunnel: w307 -> [w312 w314]
          tunnel: [w311 w313] -> w306
          frame "Idle", Default {
            n99 = call <vilib>:"Unset Busy.vi"("error in (no error)"=w312) -> ("error out"=w311:errorcluster)  [unwired: 10 in]
          }
          frame "Busy" {
            n100 = call <vilib>:"Set Busy.vi"("error in (no error)"=w314) -> ("error out"=w313:errorcluster)  [unwired: 9 in, 1 out]
          }
        }
        n101 = call <vilib>:"Add State(s) to Queue__JKI_lib_State_Machine.vi"("State(s) in (\"\")"=w310) -> ("States Out"=w309:string)  [unwired: 14 in]
      }
      frame "UI: Front Panel State" {
        # "Argument"
        # "Set Front Panel Open or Closed\n(Usage: \"UI: Front Panel State >> Open|Close\")"
        n102 = Unbundle By Name(w319) -> ("Core.Current VI Reference"=w318:refnum<vi>)
        n103 = case shown="\"Minimize\", \"Minimized\"" w317 {
          tunnel: w321 -> [w329 w344 w355 w368 w381]
          tunnel: [w331 w345 w357 w370 w383] -> w320
          tunnel: w318 -> [w330 w342 w356 w369 w382]
          frame "Open", "Standard", Default {
            w324 = T2."Standard" ("State")
            n104 = property class="VI"(reference=w330, error in=w329) -> (reference out=w327:refnum<vi>, error out=w328:errorcluster, "FP.State"=w326:T2)
            n105 = Not Equal?(x=w326, y=w324) -> (x != y?=w325:bool)
            n106 = case shown="True" w325 {
              tunnel: [w335 w337] -> w331
              tunnel: w328 -> [w334 w337]
              tunnel: w327 -> [w333 _]
              tunnel: w324 -> [w332 _]
              frame True {
                n107 = invoke class="VI" method="FP.Open"(reference=w333, error in=w334, "Activate"=TRUE, "State"=w332) -> (error out=w335:errorcluster)  [unwired: 1 in, 4 out]
              }
              frame False {
              }
            }
          }
          frame "Close", "Closed" {
            n108 = property class="VI"(reference=w342, error in=w344) -> (reference out=w341:refnum<vi>, error out=w343:errorcluster, "FP.State"=w339:T2)
            n109 = Not Equal?(x=w339, y=T2."Closed" ("Front Panel Window:State")) -> (x != y?=w338:bool)
            n110 = case shown="True" w338 {
              tunnel: [w346 w349] -> w345
              tunnel: w343 -> [w346 w348]
              tunnel: w341 -> [_ w347]
              frame False {
              }
              frame True {
                n111 = invoke class="VI" method="FP.Close"(reference=w347, error in=w348) -> (error out=w349:errorcluster)  [unwired: 1 in, 2 out]
              }
            }
          }
          frame "Hidden", "Hide" {
            w350 = T2."Hidden" ("State")
            n112 = property class="VI"(reference=w356, error in=w355) -> (reference out=w353:refnum<vi>, error out=w354:errorcluster, "FP.State"=w352:T2)
            n113 = Not Equal?(x=w352, y=w350) -> (x != y?=w351:bool)
            n114 = case shown="True" w351 {
              tunnel: [w361 w362] -> w357
              tunnel: w354 -> [w360 w362]
              tunnel: w353 -> [w359 _]
              tunnel: w350 -> [w358 _]
              frame True {
                n115 = invoke class="VI" method="FP.Open"(reference=w359, error in=w360, "State"=w358) -> (error out=w361:errorcluster)  [unwired: 2 in, 4 out]
              }
              frame False {
              }
            }
          }
          frame "Minimize", "Minimized" {
            w363 = T2."Minimized" ("State")
            n116 = property class="VI"(reference=w369, error in=w368) -> (reference out=w366:refnum<vi>, error out=w367:errorcluster, "FP.State"=w365:T2)
            n117 = Not Equal?(x=w365, y=w363) -> (x != y?=w364:bool)
            n118 = case shown="True" w364 {
              tunnel: [w374 w375] -> w370
              tunnel: w367 -> [w373 w375]
              tunnel: w366 -> [w372 _]
              tunnel: w363 -> [w371 _]
              frame True {
                n119 = invoke class="VI" method="FP.Open"(reference=w372, error in=w373, "State"=w371) -> (error out=w374:errorcluster)  [unwired: 2 in, 4 out]
              }
              frame False {
              }
            }
          }
          frame "Maximize", "Maximized" {
            w376 = T2."Maximized" ("State")
            n120 = property class="VI"(reference=w382, error in=w381) -> (reference out=w379:refnum<vi>, error out=w380:errorcluster, "FP.State"=w378:T2)
            n121 = Not Equal?(x=w378, y=w376) -> (x != y?=w377:bool)
            n122 = case shown="True" w377 {
              tunnel: [w387 w388] -> w383
              tunnel: w380 -> [w386 w388]
              tunnel: w379 -> [w385 _]
              tunnel: w376 -> [w384 _]
              frame True {
                n123 = invoke class="VI" method="FP.Open"(reference=w385, error in=w386, "State"=w384) -> (error out=w387:errorcluster)  [unwired: 2 in, 4 out]
              }
              frame False {
              }
            }
          }
        }
        n124 = call <vilib>:"Add State(s) to Queue__JKI_lib_State_Machine.vi"("State(s) in (\"\")"=w323) -> ("States Out"=w322:string)  [unwired: 14 in]
      }
      frame "UI: Resize Dashboard" {
        # "Do not put any code in this frame.\n(It is a separator no-op. You can make a copy of this frame to create a new UI frame)"
        n125 = control-ref of="Dashboard"() -> (w398:refnum<vi>)
        n126 = control-ref of="Pane 3"() -> (w391:refnum<vi>)
        n127 = Unbundle By Name(w396) -> ("NumCols"=w394:i16, "NumRows"=w395:i16)
        n128 = property class="Pane"(reference=w391) -> ("Width"=w390:u32, "Height"=w389:u32)  [unwired: 1 in, 2 out]
        n129 = call "Dashboard Cell2 Array Resize.vi"("Num Columns"=w394, "Num Rows"=w395, "area height"=w389, "area width"=w390, "Array 2"=w398) -> ("error out"=w397:errorcluster)  [unwired: 6 in]
        n130 = call <vilib>:"Add State(s) to Queue__JKI_lib_State_Machine.vi"("State(s) in (\"\")"=w400) -> ("States Out"=w399:string)  [unwired: 14 in]
      }
      frame "UI: Update Dashboard" {
        # "Do not put any code in this frame.\n(It is a separator no-op. You can make a copy of this frame to create a new UI frame)"
        n131 = Get Variant Attribute(Variant=w406) -> (duplicate Variant=w407:variant, names=w405:string[], values=w404:variant[])  [unwired: 3 in, 1 out]
        n132 = Variant To Data(type=T4[] [], Variant=w404) -> (data=w401:T4[])  [unwired: 1 in, 1 out]
        n133 = for {
          tunnel: w405 -> [w420] mode=indexing
          tunnel: [w419] -> w411 mode=indexing
          tunnel: w401 -> [w418] mode=indexing
          n134 = Unbundle By Name(w418) -> ("Current State"=w417:string, "Arguments"=w416:string)  [unwired: 1 out]
          n135 = Bundle By Name(cluster=T6 {"Label"="", "Value"="", "String"=""}, "Label"=w420, "Value"=w417, "String"=w416) -> (w419:T6)
        }
        n136 = Unbundle By Name(w412) -> ("NumRows"=w409:i16, "NumCols"=w408:i16)
        n137 = Reshape Array(w411, w409, w408) -> (→"Dashboard":T1)
        n138 = call <vilib>:"Add State(s) to Queue__JKI_lib_State_Machine.vi"("State(s) in (\"\")"=w415) -> ("States Out"=w414:string)  [unwired: 14 in]
      }
      frame "UI: Update Column Names" {
        n139 = Unbundle By Name(w423) -> ("JKISM Names"=w422:string[])
        n140 = property on="Table Control" class="Tbl (strict)"("Column Headers[]"=w422) -> ()  [unwired: 2 in, 2 out]
      }
      frame "--------- Event ---------" {
      }
      frame "Register User Event" {
        n141 = call "CSM - Global Log Event.vi"() -> ("Error out"=w436:errorcluster, "CSM Global Log Event"=w433:refnum<user-event>)  [unwired: 10 in]
        n142 = register-events(error in=w436, w433) -> (reference out=w435:refnum<event-registration>)  [unwired: 1 in, 1 out]
        n143 = Bundle By Name(cluster=w438, "CSM Global Log Event"=w433) -> (w434:T7)
      }
      frame "UnRegister User Event" {
        n144 = Unregister For Events(event registration refnum=w445) -> (error out=w444:errorcluster)  [unwired: 1 in]
        n145 = Unbundle By Name(w443) -> ("CSM Global Log Event"=w442:refnum<user-event>)
        n146 = call "CSM - Destroy Global Log Event.vi"("Error in"=w444, "CSM Global Log Event"=w442) -> ("Error out"=w441:errorcluster)  [unwired: 9 in]
        n147 = call <vilib>:"Clear Errors.vi"("error in (no error)"=w441) -> ()  [unwired: 5 in, 2 out]
      }
      frame "---------- Macro ----------" {
        # "Do not put any code in this frame.\n(It is a separator no-op. You can make a copy of this frame to create a new Macro frame)"
        n148 = call <vilib>:"Add State(s) to Queue__JKI_lib_State_Machine.vi"("State(s) in (\"\")"=w454) -> ("States Out"=w453:string)  [unwired: 14 in]
      }
      frame "Macro: Initialize" {
        # "Initialization Macro\n(This is called once, when the VI starts)"
        n149 = call <vilib>:"Add State(s) to Queue__JKI_lib_State_Machine.vi"("State(s) in Front (\"\")"="Data: Initialize\nInitialize Core Data\nData: Load from INI\nUI: Initialize\nUI: Resize Dashboard\nRegister User Event\n//UI: Front Panel State >> Open", "State(s) in (\"\")"=w461) -> ("States Out"=w460:string)  [unwired: 13 in]
      }
      frame "Macro: UI Refresh" {
        # "Do not put any code in this frame.\n(It is a separator no-op. You can make a copy of this frame to create a new Macro frame)"
        n150 = call <vilib>:"Add State(s) to Queue__JKI_lib_State_Machine.vi"("State(s) at Back (\"\")"="Macro: Update Terminal UI" ("State(s) in Front (\"\")")) -> ("States Out"=w466:string)  [unwired: 14 in]
        n151 = call <vilib>:"Add State(s) to Queue__JKI_lib_State_Machine.vi"("State(s) in Front (\"\")"=w466, "State(s) in (\"\")"=w469) -> ("States Out"=w468:string)  [unwired: 13 in]
      }
      frame "Macro: Update Terminal UI" {
        # "Do not put any code in this frame.\n(It is a separator no-op. You can make a copy of this frame to create a new Macro frame)"
        n152 = call <vilib>:"Add State(s) to Queue__JKI_lib_State_Machine.vi"("State(s) in Front (\"\")"="UI: Update Dashboard" ("State(s) in Front (\"\")"), "State(s) in (\"\")"=w476) -> ("States Out"=w475:string)  [unwired: 13 in]
      }
      frame "Macro: Exit" {
        # "Exit Macro\n(This is called once, when the VI exits)"
        n153 = Unbundle By Name(w486) -> ("Core.Close Panel on Exit?"=w485:bool)
        n154 = Select(t="UI: Front Panel State >> Close", s=w485, f="") -> (s? t:f=w481:string)
        n155 = call <vilib>:"Add State(s) to Queue__JKI_lib_State_Machine.vi"("State(s) in Front (\"\")"="UnRegister User Event" ("State(s) in Front (\"\")"), "State(s) in (\"\")"=w481, "State(s) at Back (\"\")"="Data: Save to INI\nData: Cleanup\nExit") -> ("States Out"=w484:string)  [unwired: 12 in]
        n156 = call <vilib>:"Add State(s) to Queue__JKI_lib_State_Machine.vi"("State(s) in Front (\"\")"=w484, "State(s) in (\"\")"=w489) -> ("States Out"=w488:string)  [unwired: 13 in]
      }
      frame "----- Action ------" {
      }
      frame "Action: Clear Non-exist JKISM" {
        n157 = Get Variant Attribute(Variant=w501) -> (duplicate Variant=w500:variant, names=w498:string[], values=w497:variant[])  [unwired: 3 in, 1 out]
        n158 = Variant To Data(type=T4[] [], Variant=w497) -> (data=w496:T4[])  [unwired: 1 in, 1 out]
        n159 = for {
          shift-right: [w517] -> w499
          shift-left: w500 -> [w518]
          tunnel: w498 -> [w516] mode=indexing
          tunnel: w496 -> [w515] mode=indexing
          n160 = Unbundle By Name(w515) -> ("Current State"=w513:string, "Name(\"\" to use uuid)"=w512:string)
          n161 = Search 1D Array(1D array=string[] ["<Remaining States>", "Exit"], element=w513) -> (index of element=w509:i32)  [unwired: 1 in]
          n162 = Match Pattern(string=w512, regular expression="^-") -> (offset past match=w510:i32)  [unwired: 1 in, 3 out]
          n163 = Greater Or Equal To 0?(x=w509) -> (x >= 0?=w507:bool)
          n164 = Greater Or Equal To 0?(x=w510) -> (x >= 0?=w508:bool)
          n165 = Or(x=w508, y=w507) -> (x .or. y?=w506:bool)
          n166 = case shown="True" w506 {
            tunnel: w518 -> [w519 w522]
            tunnel: [w519 w521] -> w517
            tunnel: w516 -> [_ w520]
            tunnel: w512 -> [_ _]
            tunnel: w513 -> [_ _]
            frame False {
            }
            frame True {
              n167 = Delete Variant Attribute(6:w520, 7:w522) -> (3:w521:variant)  [unwired: 1 in, 2 out]
            }
          }
        }
      }
    }
  }
